vi "Load IQ samples to memo.vi"(6 "wr.start addr":u32, 7 "burst memo":T1, 9 "wr.enable":bool, 11 "DRAM resources":T2={"DRAM read data FIFO"="", "DRAM write data FIFO"="", "DRAM request FIFO"="", "DRAM U512 memo"=refnum, "DMA data loader"="custom data", "BRAM read data FIFO"="", "BRAM write data FIFO"="", "BRAM request FIFO"="", "BRAM U512 memo"=refnum}) -> ()   [LabVIEW 2019, in "TX burst sequencer.lvlib"]
doc: "Reads data from Loader DMA as 16 samples of U32 and enques them to DRAM write fifo along with write addres. \n\nData is written sequentially from <b>wr.start addr</b> after rising edge on <b>wr.enable</b>"
uses:
  DRAM resources.ctl
  <instrlib>/_niInstr/Memory/v1/FPGA/DRAM U512/niInstr Memory DRAM U512 v1 FPGA.lvclass
  <instrlib>/_niInstr/Memory/v1/FPGA/BRAM U512/niInstr Memory BRAM U512 v1 FPGA.lvclass
  Burst memo.ctl
  <vilib>/rvi/DataTransferAndStorage/Container/Common/niFpgaContainerExecOnDevCompGetState.vi
  <vilib>/rvi/Emulation/niFpgaEmulationIsFPGAContextNoSignature.vi
  <vilib>/rvi/Emulation/niFpgaSctlEmulationGetInTimedLoop.vi
  <vilib>/rvi/errors/niFpgaSetErrorForExecOnDevCompSimple.vi
  <vilib>/rvi/eio/common/nirviEmuReportErrorAndStop.vi
  <vilib>/rvi/DataTransferAndStorage/Container/Common/niFpgaContainerGetUniqueNameForEmu.vi
  <vilib>/rvi/FIFO/Fifo_Resource/nirvififoEmulationSetSize.vi
  <vilib>/rvi/FIFO/Fifo_Resource/nirviFifoEmulationQueueMgr.vi
  <instcachedir>/0/nirviFifoEmulationQueueMgr_E5CAEC123FF24DC58D834DCA3CDAA9B5.lvgen/nirviFifoEmulationQueueMgr_E5CAEC123FF24DC58D834DCA3CDAA9B5_017.vi
  <vilib>/rvi/FIFO/Fifo_Resource/nirvififoEmulationDetermineInputValidOut.vi
  <vilib>/rvi/FIFO/Fifo_Resource/nirvififoEmulationCreateLock.vi
  <vilib>/rvi/Emulation/niFpgaProcessEmulError.vi
  <vilib>/rvi/FIFO/Fifo_Resource/nirvififoEmulationObtainLock.vi
  <vilib>/rvi/FIFO/Fifo_Resource/nirvififoEmulationReleaseLock.vi
  <vilib>/rvi/occurrence/nirviWaitOnOccurrenceBase.vi
  <vilib>/rvi/errors/nirviReportUnexpectedCaseInternalError.vi
  <vilib>/rvi/errors/nirviReportUnexpectedCaseInternalError (U32).vi
  <vilib>/Utility/error.llb/Clear Errors.vi
  <vilib>/rvi/interface/RandomDataEmulation/niFpgaRandomDataHandleErrors.vi
  <vilib>/rvi/interface/RandomDataEmulation/nirviRandomDataAcquireLock.vi
  <vilib>/rvi/interface/RandomDataEmulation/nirviRandomDataQueueStore.vi
  <vilib>/rvi/interface/RandomDataEmulation/nirviRandomDataReleaseLock.vi
  <vilib>/rvi/interface/RandomDataEmulation/nirviFPGAContextMergeError.vi
  <vilib>/rvi/interface/RandomDataEmulation/nirviRandomDataCheckExitLoopConditions.vi
  <vilib>/express/rvi/timingcommon/nirviCommon.vi
  <instrlib>/_niInstr/Data Formatting/v1/FPGA/Private/Convert/FXP(+-,14,1) array to Boolean Array.vi
  <vilib>/rvi/DataTransferAndStorage/Container/XNode/niFpgaContainer.xnode
  <vilib>/rvi/FIFO/Fifo_Resource/niFpgaFifoEmulationRefIn.vi
  <vilib>/rvi/FIFO/Fifo_Resource/niFpgaFifoEmulationRefInMultiElement.vi
  TX burst sequencer.lvlib
  <instrlib>/_niInstr/Basic Elements/v1/FPGA/niInstr Basic Elements v1 FPGA.lvlib
  Utility/FPGA Utility.lvlib
  <instrlib>/_niInstr/Data Formatting/v1/FPGA/niInstr Data Formatting v1 FPGA.lvlib
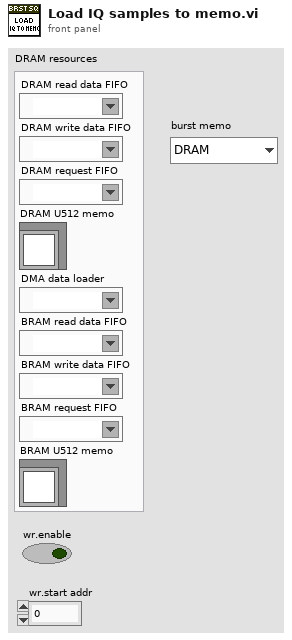
[diagram p1: front panel]
types:
  T1 = typedef "TX burst sequencer.lvlib/Burst memo.ctl" = enum16{"DRAM", "BRAM"}
  T2 = typedef "TX burst sequencer.lvlib/DRAM resources.ctl" = cluster{"DRAM read data FIFO":refnum<k21>, "DRAM write data FIFO":refnum<k21>, "DRAM request FIFO":refnum<k21>, "DRAM U512 memo":refnum<class "niInstr Memory DRAM U512 v1 FPGA.lvclass">, "DMA data loader":refnum<k21>, "BRAM read data FIFO":refnum<k21>, "BRAM write data FIFO":refnum<k21>, "BRAM request FIFO":refnum<k21>, "BRAM U512 memo":refnum<class "niInstr Memory BRAM U512 v1 FPGA.lvclass">}
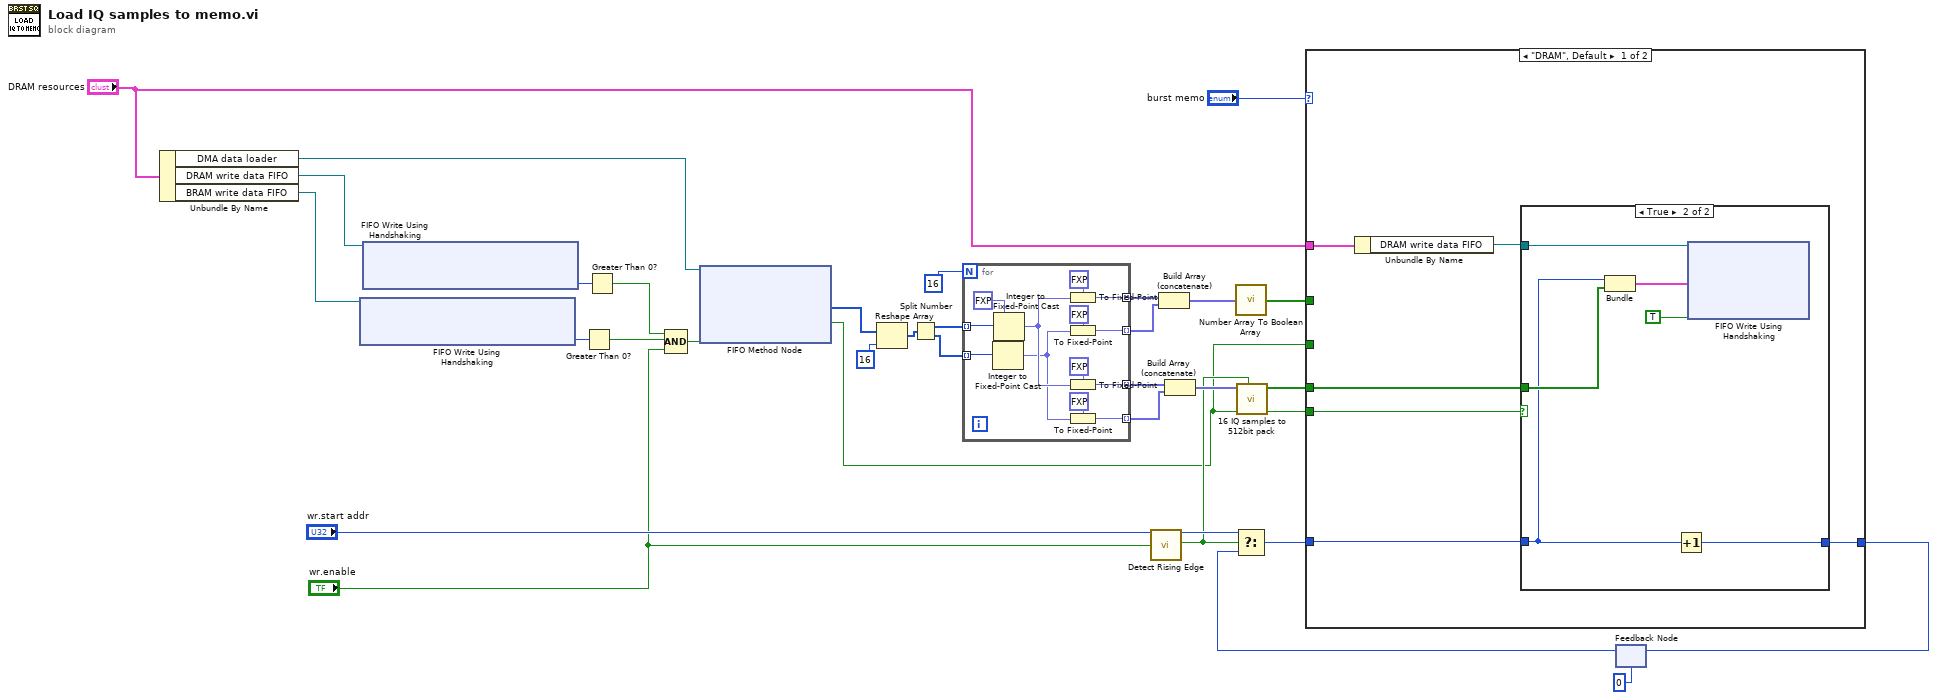
[diagram p0: block diagram]
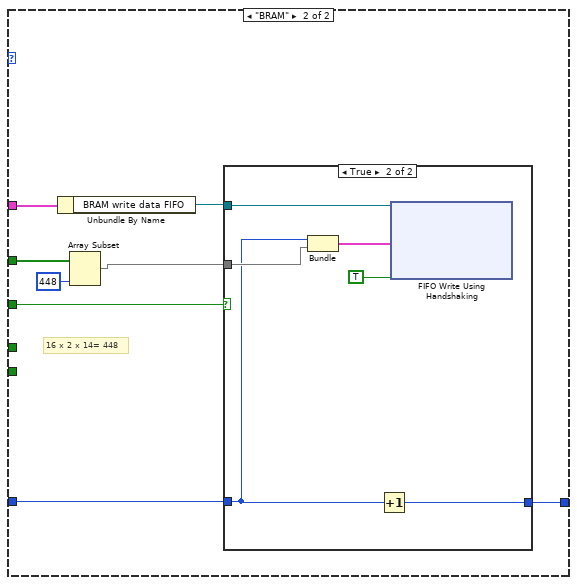
[diagram p3: hidden frame]
diagram:
  n1 = Unbundle By Name("DRAM resources") -> ("DMA data loader"=w23:refnum<k21>, "DRAM write data FIFO"=w24:refnum<k21>, "BRAM write data FIFO"=w8:refnum<k21>)
  n2 = xnode ("FIFO Write Using Handshaking")("FIFO In"=w8) -> ("Number of Elements to Write"=w7:u32)  [unwired: 1 out]
  n3 = xnode ("FIFO Write Using Handshaking")("FIFO In"=w24) -> ("Number of Elements to Write"=w31:u32)  [unwired: 1 out]
  n4 = Greater Than 0?(x=w7) -> (x > 0?=w6:bool)
  n5 = Greater Than 0?(x=w31) -> (x > 0?=w33:bool)
  n6 = Compound Arithmetic op=AND(w33, w6, "wr.enable") -> (w32:bool)
  n7 = xnode ("FIFO Method Node")("Ready for Output"=w32, "FIFO In"=w23) -> ("Element"=w18:u32[], "Output Valid"=w2:bool)  [unwired: 1 out]
  n8 = Reshape Array(w18, 16 ("dimension size")) -> (w21:u32[])
  n9 = Split Number(x=w21) -> (hi(x)=w20:u16[], lo(x)=w19:u16[])
  n10 = for {
    N: 16 -> [_]
    tunnel: w20 -> [w46] mode=indexing
    tunnel: w19 -> [w45] mode=indexing
    tunnel: [w41] -> w16 mode=indexing
    tunnel: [w40] -> w15 mode=indexing
    tunnel: [w35] -> w10 mode=indexing
    tunnel: [w34] -> w11 mode=indexing
    w44 = fxp<+/-,16,1> 0.0 ("fixed-point type")
    n11 = Integer to Fixed-Point Cast(fixed-point type=w44, integer=w45) -> (fixed-point=w36:fxp<+/-,16,1>)
    n12 = Integer to Fixed-Point Cast(fixed-point type=w44, integer=w46) -> (fixed-point=w39:fxp<+/-,16,1>)
    n13 = To Fixed-Point(fixed-point type=fxp<+/-,14,1> 0.0, number=w39) -> (fixed-point=w34:fxp<+/-,14,1>)
    n14 = To Fixed-Point(fixed-point type=fxp<+/-,14,1> 0.0, number=w36) -> (fixed-point=w35:fxp<+/-,14,1>)
    n15 = To Fixed-Point(fixed-point type=fxp<+/-,12,1> 0.0, number=w39) -> (fixed-point=w41:fxp<+/-,12,1>)
    n16 = To Fixed-Point(fixed-point type=fxp<+/-,12,1> 0.0, number=w36) -> (fixed-point=w40:fxp<+/-,12,1>)
  }
  n17 = call <instrlib>:"Detect Rising Edge.vi"("signal"="wr.enable") -> ("edge detected"=w13:bool)  [unwired: 14 in]
  n18 = Build Array (concatenate)(w11, w10) -> (w9:fxp<+/-,14,1>[])
  n19 = Build Array (concatenate)(w16, w15) -> (w14:fxp<+/-,12,1>[])
  n20 = call-poly <instrlib>:"Number Array To Boolean Array.vi"("data in"=w9) -> ("data out"=w3:bool[])  [unwired: 14 in]
  n21 = call "16 IQ samples to 512bit pack.vi"("reset"=w13, "input valid"=w2, "data in"=w14) -> ("output valid"=w12:bool, "data out"=w1:bool[])  [unwired: 6 in, 1 out]
  n22 = feedback #1(u32 0) -> (w29:u32)
  n23 = Select(t="wr.start addr", s=w13, f=w29) -> (s? t:f=w27:u32)
  n24 = case shown="\"DRAM\", Default" "burst memo" {
    tunnel: [w52 w67] -> w28
    tunnel: w27 -> [w51 w66]
    tunnel: w12 -> [w50 _]
    tunnel: "DRAM resources" -> [w49 w65]
    tunnel: w3 -> [_ w62]
    tunnel: w2 -> [_ w63]
    tunnel: w1 -> [w47 _]
    frame "DRAM", Default {
      n25 = Unbundle By Name(w49) -> ("DRAM write data FIFO"=w48:refnum<k21>)
      n26 = case shown="True" w50 {
        tunnel: w47 -> [_ w58]
        tunnel: w48 -> [_ w59]
        tunnel: w51 -> [w53 w55]
        tunnel: [w53 w54] -> w52
        frame False {
        }
        frame True {
          n27 = Bundle("wr.start addr"=w55, "data out"=w58) -> (w57:cluster{"wr.start addr":u32, "data out":bool[]})  [unwired: 1 in]
          n28 = Increment(x=w55) -> (x+1=w54:u32)
          n29 = xnode ("FIFO Write Using Handshaking")("Element"=w57, "Input Valid"=TRUE, "FIFO In"=w59) -> ()  [unwired: 2 out]
        }
      }
    }
    frame "BRAM" {
      # "16 x 2 x 14= 448"
      n30 = Unbundle By Name(w65) -> ("BRAM write data FIFO"=w64:refnum<k21>)
      n31 = Array Subset(array=w62, length=448) -> (w60:bool[])  [unwired: 1 in]
      n32 = case shown="True" w63 {
        tunnel: w60 -> [_ w73]
        tunnel: w64 -> [_ w74]
        tunnel: w66 -> [w68 w70]
        tunnel: [w68 w69] -> w67
        frame False {
        }
        frame True {
          n33 = Bundle("wr.start addr"=w70, w73) -> (w72:cluster{"wr.start addr":u32, bool[]})  [unwired: 1 in]
          n34 = Increment(x=w70) -> (x+1=w69:u32)
          n35 = xnode ("FIFO Write Using Handshaking")("Element"=w72, "Input Valid"=TRUE, "FIFO In"=w74) -> ()  [unwired: 2 out]
        }
      }
    }
  }
  n36 = feedback-in #1(w28) -> ()
